vi "new_document.vi"(11 "Name":string) -> (1 "path":string, 2 "payload":string, 3 "Method":string)   [LabVIEW 2019]
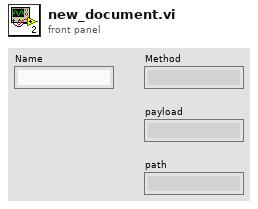
[diagram p1: front panel]
types:
  T1 = cluster{"name":string, "ownerType":i32, "isPublic":bool}
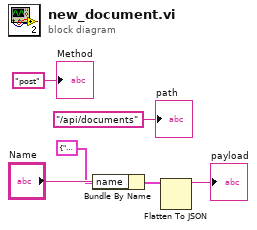
[diagram p0: block diagram]
diagram:
  n1 = Bundle By Name(cluster=T1 {"name"="milan", "ownerType"=0, "isPublic"=FALSE}, "name"="Name") -> (w4:T1)
  n2 = Flatten To JSON(anything=w4) -> (JSON string=→"payload":string)  [unwired: 2 in, 1 out]
  "path" <- "/api/documents" ("payload")
  "Method" <- "post" ("Method")
